vi "Archive Command Data.vi"(8 "error in":errorcluster, 10 "LBCB Filter":T2, 11 "Command Data":T1) -> (0 "error out":errorcluster, 2 "string":string)   [LabVIEW 2009]
uses:
  Data Access Objects/Metadata/LBCB Filter.ctl
  Target Data.ctl
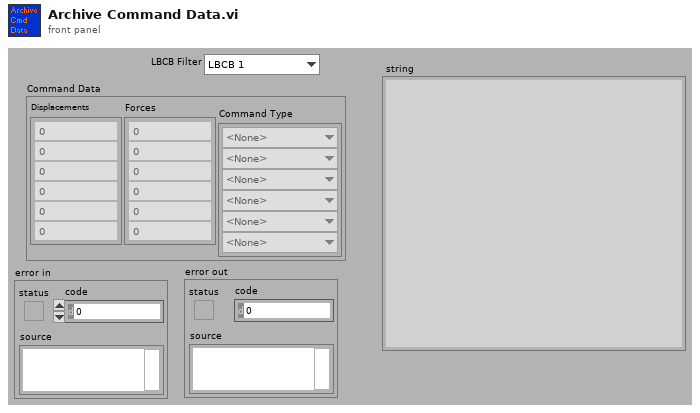
[diagram p1: front panel]
types:
  T1 = typedef "Target Data.ctl" = cluster{"Displacements":dbl[], "Command Type":enum16{"<None>", "Displacement", "Force"}[], "Forces":dbl[]}
  T2 = typedef "LBCB Filter.ctl" = enum16{"LBCB 1", "LBCB 2", "Both"}
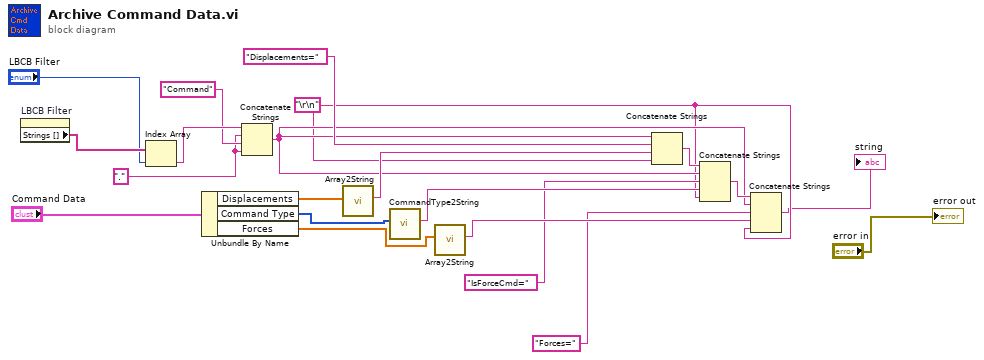
[diagram p0: block diagram]
diagram:
  w6 = "\r\n"
  w1 = "." ("string")
  n1 = property on="LBCB Filter" class="Enum (strict)"() -> ("Strings []"=w21:string[])  [unwired: 2 in, 2 out]
  n2 = Index Array(array=w21, index="LBCB Filter") -> (element=w4:string)
  n3 = Unbundle By Name("Command Data") -> ("Displacements"=w17:dbl[], "Command Type"=w18:enum16{"<None>", "Displacement", "Force"}[], "Forces"=w19:dbl[])
  n4 = Concatenate Strings(w4, w1, "Command" ("string"), w1) -> (w12:string)
  n5 = call "Array2String.vi"("Array"=w17) -> ("String"=w13:string)  [unwired: 1 in, 9 out]
  n6 = call "CommandType2String.vi"("Command\nType"=w18) -> ("String"=w11:string)  [unwired: 10 out]
  n7 = call "Array2String.vi"("Array"=w19) -> ("String"=w10:string)  [unwired: 1 in, 9 out]
  n8 = Concatenate Strings(w12, "Displacements=", w13, w6) -> (w15:string)
  n9 = Concatenate Strings(w15, w12, "IsForceCmd=", w11, w6) -> (w16:string)
  n10 = Concatenate Strings(w16, w12, "Forces=", w10, w6) -> (→"string":string)
  "error out" <- "error in"
